vi "read_active_item.vi"(8 "error in (no error)":errorcluster, 11 "StringList in":refnum<class "StringList.lvclass">) -> (0 "error out":errorcluster, 2 "List Item":string, 3 "StringList out":refnum<class "StringList.lvclass">)   [LabVIEW 2015, in "StringList.lvlib" / "StringList.lvclass"]
uses:
  StringList.lvclass
  StringList.lvclass/StringList.ctl
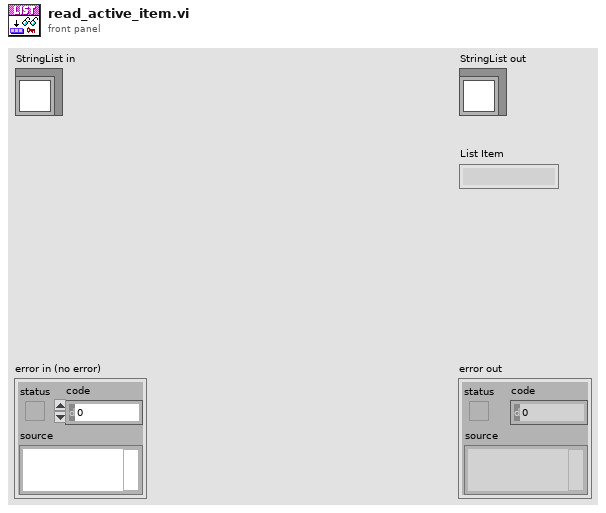
[diagram p1: front panel]
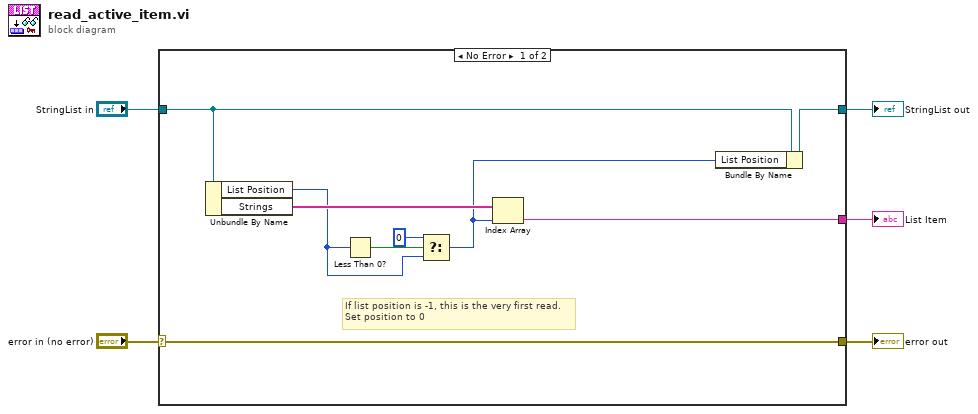
[diagram p0: block diagram]
diagram:
  n1 = case shown="No Error" "error in (no error)" {
    selector: "error in (no error)" -> [w14 w16]
    tunnel: [w14 w16] -> w4
    tunnel: [w12 w15] -> w2
    tunnel: "StringList in" -> [w13 w15]
    tunnel: [w7 _] -> w1
    frame No Error {
      # "If list position is -1, this is the very first read.\nSet position to 0"
      n2 = Unbundle By Name(w13) -> ("List Position"=w9:i32, "Strings"=w11:string[])
      n3 = Less Than 0?(x=w9) -> (x < 0?=w10:bool)
      n4 = Select(t=0, s=w10, f=w9) -> (s? t:f=w6:i32)
      n5 = Index Array(array=w11, index=w6) -> (element=w7:string)
      n6 = Bundle By Name(cluster=w13, "List Position"=w6) -> (w12:refnum<class "StringList.lvclass">)
    }
    frame Error {
    }
  }
  "error out" <- w4
  "StringList out" <- w2
  "List Item" <- w1
